vi "2D Array Statistics.vi"(2 "array":dbl[][](array[numeric])) -> (1 "number of elements":i32, 5 "max":dbl, 6 "mean":dbl, 7 "min":dbl, 8 "sum":dbl)   [LabVIEW 2018]
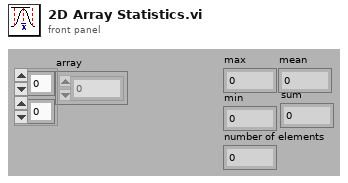
[diagram p1: front panel]
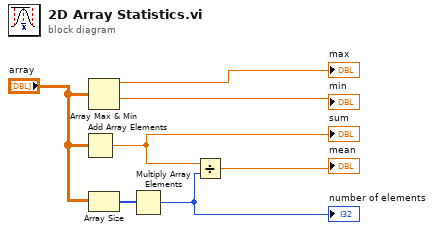
[diagram p0: block diagram]
diagram:
  n1 = Add Array Elements(numeric array="array") -> (sum=w6:dbl)
  "sum" <- w6
  n2 = Array Max & Min(array="array") -> (max value=→"max":dbl, min value=→"min":dbl)  [unwired: 2 out]
  n3 = Array Size(array="array") -> (size(s)=w5:i32[])
  n4 = Multiply Array Elements(1:w5) -> (0:w4:i32)
  "number of elements" <- w4
  n5 = Divide(x=w6, y=w4) -> (x/y=→"mean":dbl)
